vi "FiltroM2.vi"(10 "entrada":dbl, 11 "salida":dbl) -> (3 "Numeric out":dbl)   [LabVIEW 2018]
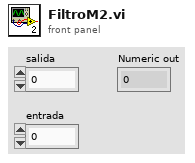
[diagram p1: front panel]
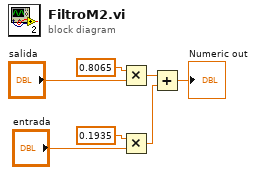
[diagram p0: block diagram]
diagram:
  n1 = Multiply(x=0.8065, y="salida") -> (x*y=w4:dbl)
  n2 = Multiply(x=0.1935, y="entrada") -> (x*y=w3:dbl)
  n3 = Add(x=w4, y=w3) -> (x+y=→"Numeric out":dbl)
